vi "InitializeResolverParameters.vi"(6 "Specified Channel Ref List":T1[](array[typedef]) format="%.0x", 8 "error in":errorcluster, 9 "FPGA Session In":refnum<class "FPGA Interface Base.lvclass">, 11 "Device Reference in":T1 format="%.0x") -> (0 "error out":errorcluster, 1 "FPGA Session Out":refnum<class "FPGA Interface Base.lvclass">, 2 "Resolver Parameters":T2[](array[typedef]), 3 "Device Reference out":T1 format="%.0x")   [LabVIEW 2011, in "Sensor Simulation Custom Device.lvlib"]
uses:
  Sensor Simulation Custom Device.lvlib
  <vilib>/NI Veristand/Custom Device API/Custom Device Item Ref.ctl
  TypeDefs/Resolver Parameters.ctl
  <userlib>/_FPGA Interface Advanced Tools/FPGA Interface Base/FPGA Interface Base.lvclass
  TypeDefs/SensorType.ctl
  System Explorer/TypeDefs/Resolver.ctl
  <vilib>/rvi/DataTransferAndStorage/Container/Common/niFpgaDataTypeControl.ctl
  <userlib>/_FPGA Interface Advanced Tools/FPGA Interface Base/FPGA Interface Base.lvclass/FPGA Interface Base.ctl
  <vilib>/NI Veristand/Custom Device Tools/Custom Device Utility Library/NI VeriStand - Search for All Items by Property.vi
  Global.vi
  <vilib>/NI Veristand/Custom Device API/Get Item Property (Variant).vi
  <vilib>/Utility/error.llb/Error Cluster From Error Code.vi
  <vilib>/NI Veristand/Custom Device API/Custom Device API.lvlib
  <vilib>/NI Veristand/Custom Device Tools/Custom Device Utility Library/Custom Device Utility Library.lvlib
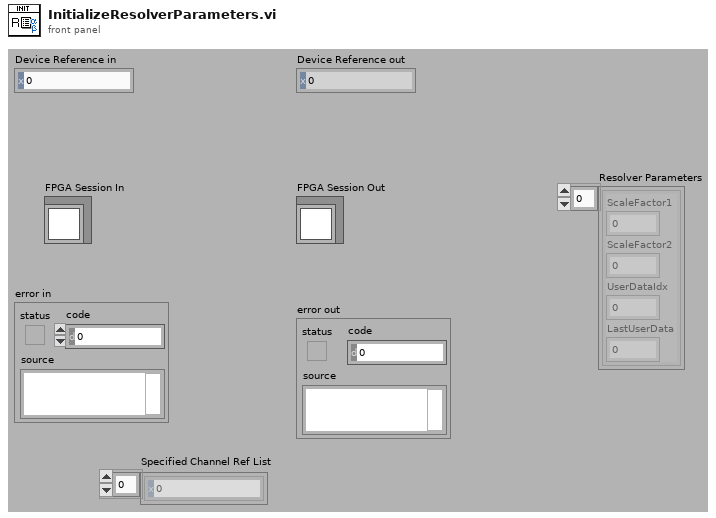
[diagram p1: front panel]
types:
  T1 = typedef "Custom Device API.lvlib/Custom Device Item Ref.ctl" = u64
  T2 = typedef "Sensor Simulation Custom Device.lvlib/Resolver Parameters.ctl" = cluster{"ScaleFactor1":u32, "ScaleFactor2":u32, "UserDataIdx":i32, "LastUserData":dbl}
  T3 = typedef "Sensor Simulation Custom Device.lvlib/SensorType.ctl" = enum16{"Resolver", "4 Wire xVDT", "5 Wire xVDT", "Invalid"}
  T4 = typedef "niFpgaDataTypeControl.ctl" = enum32{"Boolean", "I8", "I16", "I32", "I64", "U8", "U16", "U32", "U64", "FXP", "CustomControl"}
  T5 = typedef "Sensor Simulation Custom Device.lvlib/Resolver.ctl" = cluster{"ScaleFactor 1":string, "ScaleFactor 2":string, "#":string}
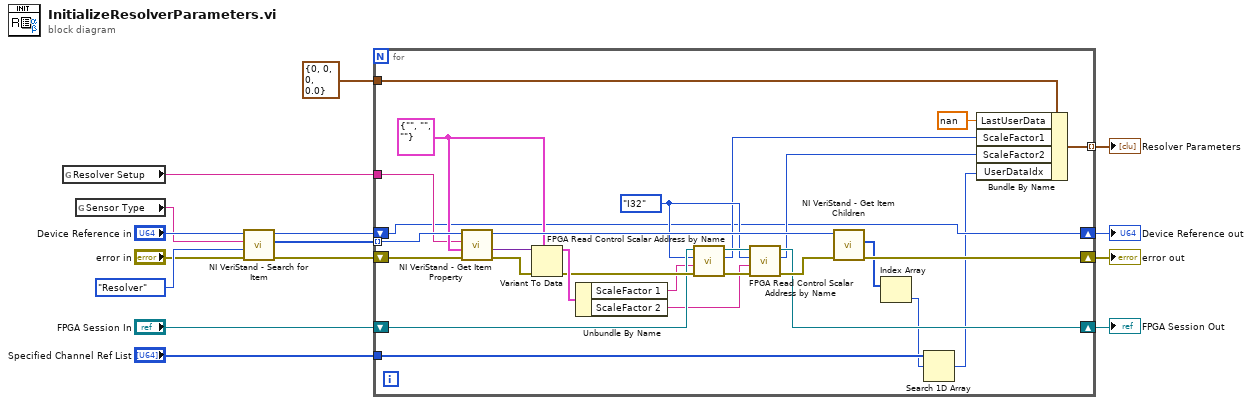
[diagram p0: block diagram]
diagram:
  n1 = global read "Global.vi" "Resolver Setup"() -> (w4:string)
  n2 = global read "Global.vi" "Sensor Type"() -> (w13:string)
  n3 = call-poly <vilib>:"NI VeriStand - Search for Item.vi"("error in"="error in", "Property Value"=SensorType."Resolver" ("Sensor"), "Property Name"=w13, "Section Ref in"="Device Reference in") -> ("error out"=w8:errorcluster, "Item Refs"=w7:T1[], "Section Ref out"=w6:T1)  [unwired: 4 in, 1 out]
  n4 = for {
    shift-right: [w22] -> w15
    shift-left: w8 -> [w37]
    tunnel: w7 -> [w36] mode=indexing
    tunnel: T2 {"ScaleFactor1"=0, "ScaleFactor2"=0, "UserDataIdx"=0, "LastUserData"=0.0} ("4 Wire LVDT Parameters") -> [w39]
    tunnel: [w38] -> w11 mode=indexing
    shift-right: [w21] -> w10
    shift-left: w6 -> [w21]
    tunnel: w4 -> [w34]
    shift-right: [w26] -> w2
    shift-left: "FPGA Session In" -> [w29]
    tunnel: "Specified Channel Ref List" -> [w19]
    w25 = niFpgaDataTypeControl."I32" ("Data Type")
    w35 = T5 {"ScaleFactor 1"="", "ScaleFactor 2"="", "#"=""}
    n5 = call-poly <vilib>:"NI VeriStand - Get Item Property.vi"("error in (no error)"=w37, "Default Value"=w35, "Property Name"=w34, "Item Ref in"=w36) -> ("error out"=w43:errorcluster, "Value"=w42:variant, "Item Ref out"=w40:T1)  [unwired: 4 in, 1 out]
    n6 = Variant To Data(error in=w43, type=w35, Variant=w42) -> (data=w41:T5, error out=w33:errorcluster)
    n7 = Unbundle By Name(w41) -> ("ScaleFactor 1"=w28:string, "ScaleFactor 2"=w27:string)
    n8 = call <userlib>:"FPGA Read Control Scalar Address by Name.vi"("error in (no error)"=w33, "Name"=w28, "Data Type"=w25, "FPGA Interface Base in"=w29) -> ("error out"=w32:errorcluster, "Address"=w24:u32, "FPGA Interface Base out"=w31:refnum<class "FPGA Interface Base.lvclass">)  [unwired: 4 in, 1 out]
    n9 = call <userlib>:"FPGA Read Control Scalar Address by Name.vi"("error in (no error)"=w32, "Name"=w27, "Data Type"=w25, "FPGA Interface Base in"=w31) -> ("error out"=w30:errorcluster, "Address"=w23:u32, "FPGA Interface Base out"=w26:refnum<class "FPGA Interface Base.lvclass">)  [unwired: 4 in, 1 out]
    n10 = call <vilib>:"NI VeriStand - Get Item Children.vi"("error in (no error)"=w30, "Item Ref in"=w40) -> ("error out"=w22:errorcluster, "Child Refs"=w20:T1[])  [unwired: 6 in, 2 out]
    n11 = Index Array(array=w20) -> (element=w18:T1)  [unwired: 1 in]
    n12 = Search 1D Array(1D array=w19, element=w18) -> (index of element=w17:i32)  [unwired: 1 in]
    n13 = Bundle By Name(cluster=w39, "LastUserData"=nan, "ScaleFactor1"=w24, "ScaleFactor2"=w23, "UserDataIdx"=w17) -> (w38:T2)
  }
  "error out" <- w15
  "Device Reference out" <- w10
  "Resolver Parameters" <- w11
  "FPGA Session Out" <- w2
